vi "Wait for Configuration.vi"(8 "error in (no error)":errorcluster, 11 "Statnett C37.118 DLL in":refnum<class "Statnett C37.118 DLL.lvclass">) -> (0 "error out":errorcluster, 3 "Statnett C37.118 DLL out":refnum<class "Statnett C37.118 DLL.lvclass">)   [LabVIEW 2013, in "PMU Recorder Light.lvlib" / "Statnett C37.118 DLL.lvclass"]
uses:
  Statnett C37.118 DLL.lvclass
  Statnett C37.118 DLL.lvclass/Statnett C37.118 DLL.ctl
  c37118-dll/labview/C37118-DLL.lvlib
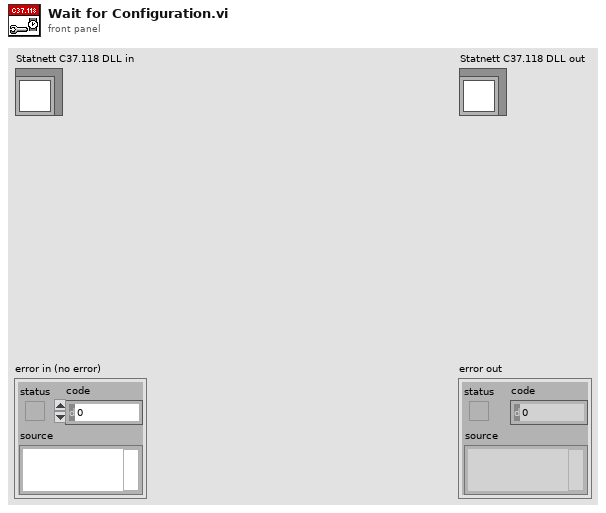
[diagram p1: front panel]
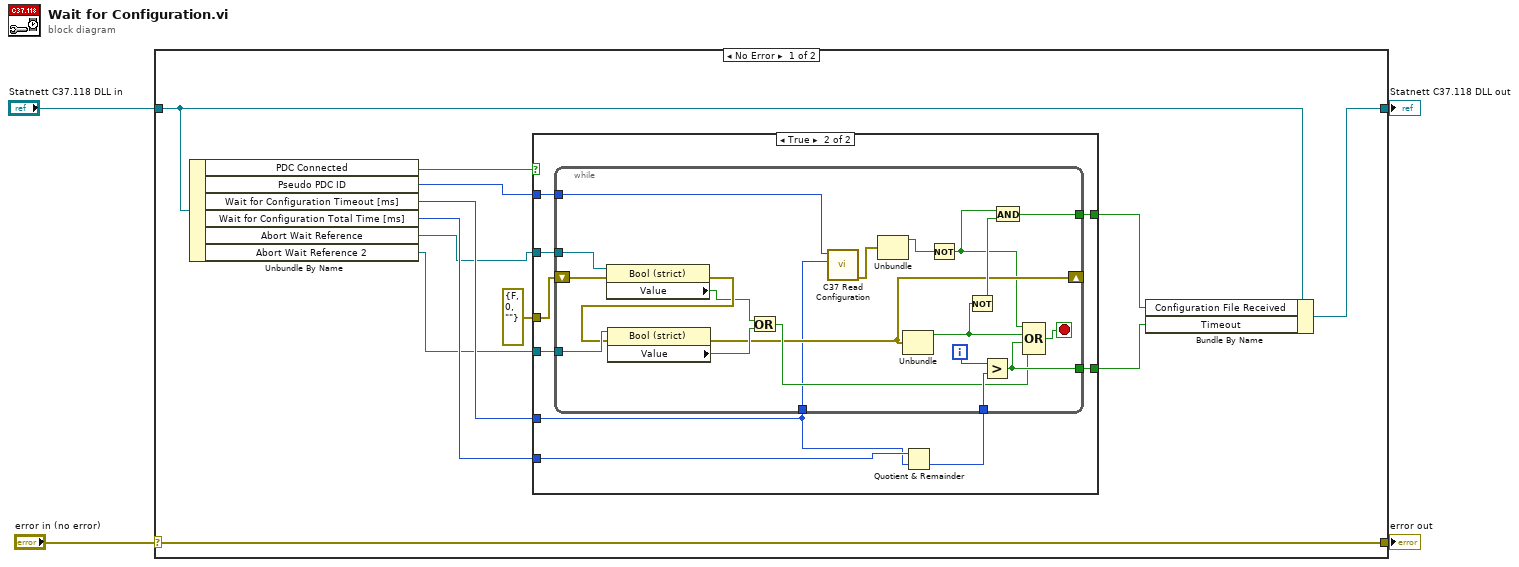
[diagram p0: block diagram]
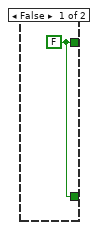
[diagram p2: hidden frame]
diagram:
  n1 = case shown="No Error" "error in (no error)" {
    selector: "error in (no error)" -> [w16 w48]
    tunnel: [w16 w48] -> w3
    tunnel: [w8 w47] -> w1
    tunnel: "Statnett C37.118 DLL in" -> [w9 w47]
    frame No Error {
      n2 = Unbundle By Name(w9) -> ("PDC Connected"=w14:bool, "Pseudo PDC ID"=w7:i32, "Wait for Configuration Timeout [ms]"=w13:i32, "Wait for Configuration Total Time [ms]"=w12:i32, "Abort Wait Reference"=w6:refnum<vi>, "Abort Wait Reference 2"=w5:refnum<vi>)
      n3 = case shown="True" w14 {
        tunnel: w6 -> [_ w25]
        tunnel: [w17 w24] -> w10
        tunnel: [w17 w23] -> w11
        tunnel: w12 -> [_ w21]
        tunnel: errorcluster {"status"=FALSE, "code"=0, "source"=""} ("error IO") -> [_ w22]
        tunnel: w13 -> [_ w20]
        tunnel: w5 -> [_ w19]
        tunnel: w7 -> [_ w18]
        frame False {
          w17 = FALSE
        }
        frame True {
          n4 = Quotient & Remainder(x=w21, y=w20) -> (floor(x/y)=w26:i32)  [unwired: 1 out]
          n5 = while {
            shift-right: [w32] -> _
            shift-left: w22 -> [w39]
            tunnel: [w43] -> w23
            tunnel: [w41] -> w24
            tunnel: w25 -> [w40]
            tunnel: w20 -> [w27]
            tunnel: w26 -> [w38]
            tunnel: w19 -> [w37]
            tunnel: w18 -> [w28]
            i -> [w42]
            stop <- w46 stop-if-true
            n6 = property class="Bool (strict)"(reference=w40, error in=w39) -> (error out=w36:errorcluster, "Value"=w35:bool)  [unwired: 1 out]
            n7 = property class="Bool (strict)"(reference=w37, error in=w36) -> (error out=w32:errorcluster, "Value"=w34:bool)  [unwired: 1 out]
            n8 = Or(x=w35, y=w34) -> (x .or. y?=w33:bool)
            n9 = call "C37 Read Configuration.vi"("Timeout [ms]"=w27, "Pseudo PDC ID"=w28) -> ("error out"=w29:errorcluster)  [unwired: 9 in]
            n10 = Unbundle(w29) -> ("status"=w30:bool)  [unwired: 2 out]
            n11 = Unbundle(w32) -> ("status"=w45:bool)  [unwired: 2 out]
            n12 = Not(x=w30) -> (.not. x?=w31:bool)
            n13 = Not(x=w45) -> (.not. x?=w44:bool)
            n14 = Greater?(x=w42, y=w38) -> (0:w41:bool)
            n15 = And(x=w31, y=w44) -> (x .and. y?=w43:bool)
            n16 = Compound Arithmetic op=OR(w31, w45, w41, w33) -> (w46:bool)
          }
        }
      }
      n17 = Bundle By Name(cluster=w9, "Configuration File Received"=w11, "Timeout"=w10) -> (w8:refnum<class "Statnett C37.118 DLL.lvclass">)
    }
    frame Error {
    }
  }
  "error out" <- w3
  "Statnett C37.118 DLL out" <- w1
